vi "cont_acquisition.vi"() -> ()   [LabVIEW 2011]
uses:
  <vilib>/vision/driver/IMAQdx.llb/IMAQdx Attribute Type.ctl
  global_vars.vi
  <vilib>/vision/driver/NI_Vision_Acquisition_Software.lvlib
panel:
  out "Attribute Information Array":T2(array[cluster])
  out "Frame Rate":dbl
  in  "Close":bool
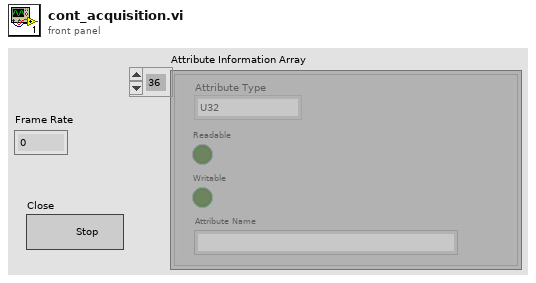
[diagram p1: front panel]
types:
  T1 = typedef "NI_Vision_Acquisition_Software.lvlib/IMAQdx Attribute Type.ctl" = enum32{"U32", "I64", "DBL", "String", "Enum", "Bool", "Command"}
  T2 = cluster{"Attribute Type":T1, "Readable":bool, "Writable":bool, "Attribute Name":string}[]
  T3 = typedef "IMAQdx.ctl" = refnum<k21>
  T4 = typedef "IMAQ Image.ctl" = refnum<image>
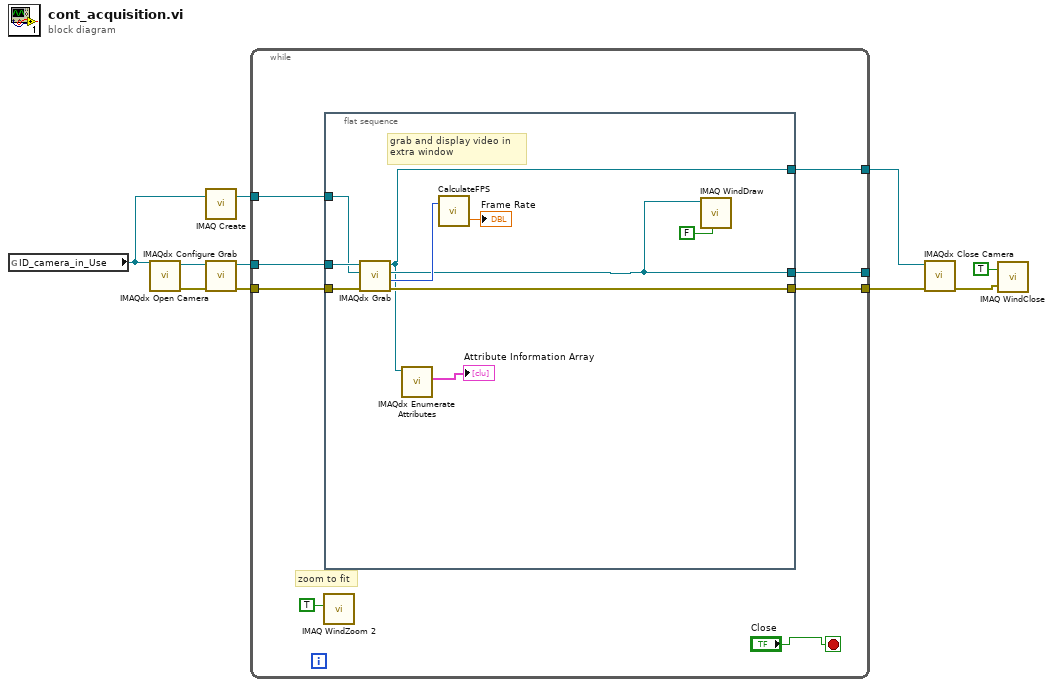
[diagram p0: block diagram]
diagram:
  n1 = global read "global_vars.vi" "ID_camera_in_Use"() -> (w2:T3)
  n2 = call <vilib>:"IMAQdx Open Camera.vi"("Session In"=w2) -> ("error out"=w6:errorcluster, "Session Out"=w5:T3)  [unwired: 2 in, 7 out]
  n3 = call "IMAQ Create"("Image Name"=w2) -> ("New Image"=w10:T4)  [unwired: 3 in, 2 out]
  n4 = call <vilib>:"IMAQdx Configure Grab.vi"("error in"=w6, "Session In"=w5) -> ("error out"=w8:errorcluster, "Session Out"=w9:T3)  [unwired: 8 out]
  n5 = while {
    tunnel: w8 -> [w17]
    tunnel: w9 -> [w18]
    tunnel: [w15] -> w7
    tunnel: w10 -> [w16]
    tunnel: [w13] -> _
    tunnel: [w12] -> w1
    stop <- "Close" stop-if-true
    # "zoom to fit"
    n6 = call "IMAQ WindZoom 2"("Zoom to Fit? (False)"=TRUE) -> ()  [unwired: 7 in, 4 out]
    n7 = flat-sequence {
      tunnel: [w25] -> w15
      tunnel: w18 -> [w28]
      tunnel: w17 -> [w27]
      tunnel: w16 -> [w26]
      tunnel: [w20] -> w13
      tunnel: [w19] -> w12
      frame #0 {
        # "grab and display video in \nextra window"
        n8 = call <vilib>:"IMAQdx Grab.vi"("error in"=w27, "Image In"=w26, "Session In"=w28) -> ("error out"=w25:errorcluster, "Buffer Number Out"=w23:u32, "Image Out"=w20:T4, "Session Out"=w19:T3)  [unwired: 1 in, 4 out]
        n9 = call <vilib>:"IMAQdx Enumerate Attributes.vi"("Session In"=w19) -> ("Attribute Information Array"=→"Attribute Information Array":T2)  [unwired: 8 in, 2 out]
        n10 = call "CalculateFPS.vi"("buffer number"=w23) -> ("processed FPS"=→"Frame Rate":dbl)  [unwired: 2 out]
        n11 = call "IMAQ WindDraw"("Resize to Image Size? (Y)"=FALSE, "Image"=w20) -> ()  [unwired: 8 in, 2 out]
      }
    }
  }
  n12 = call <vilib>:"IMAQdx Close Camera.vi"("error in"=w7, "Session In"=w1) -> ("error out"=w3:errorcluster)  [unwired: 9 out]
  n13 = call "IMAQ WindClose"("Close All Windows (False)"=TRUE, "error in (no error)"=w3) -> ()  [unwired: 4 in, 1 out]
